vi "Correlation_Display.vi"(5 "Inst names":string[](array[string])=["HW 1", "HW 2"], 6 "OK":bool) -> (2 "correlation array":i32[][](array[numeric]) min=0 max=8)   [LabVIEW 2011]
uses:
  Globals/Meas_global.vi
panel:
  in  "number of correlation pairs":i32=1
  in  "correlation choices":i32[][](array[ring])=[[0, 1], [0, 0], [0, 0]] items=["LDA (U)", "LDA (W)", "XW (U) LDA Sync", "XW (W) LDA Sync", "RV (Sync)", "XW (U)", "XW (W)", "XW  U1", "XW  U2"]
  # "1st Pair"
  # "2nd Pair"
  # "3rd Pair"
  # "4th Pair"
  # "5th Pair"
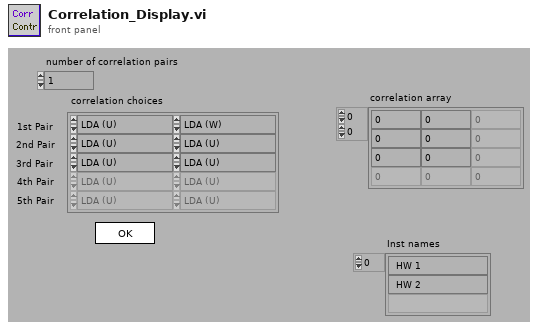
[diagram p1: front panel]
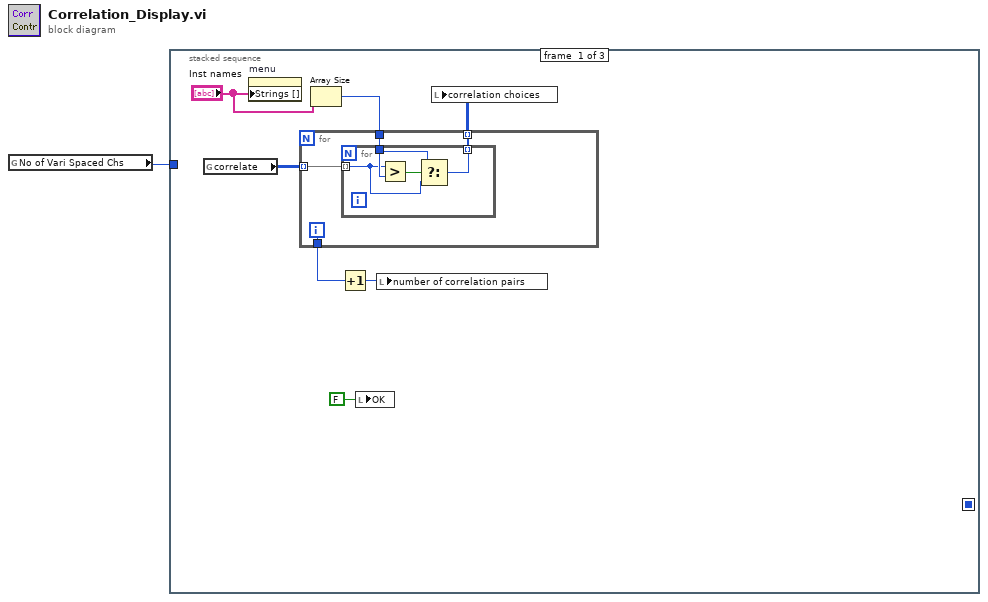
[diagram p0: block diagram]
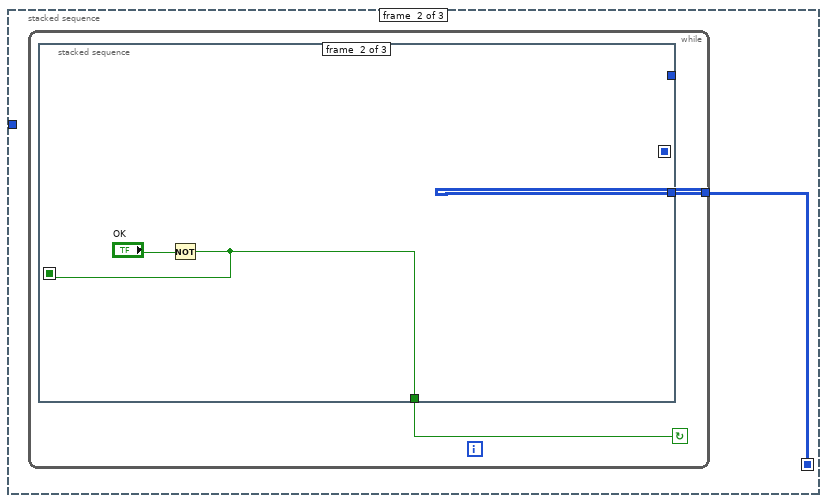
[diagram p2: hidden frame]
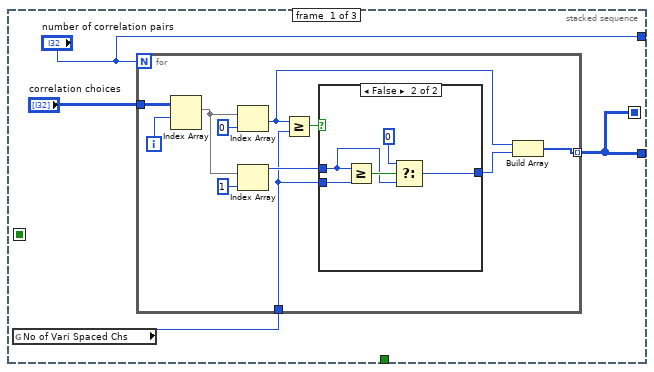
[diagram p3: hidden frame]
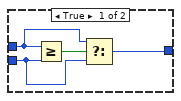
[diagram p4: hidden frame]
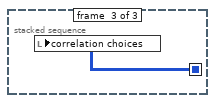
[diagram p5: hidden frame]
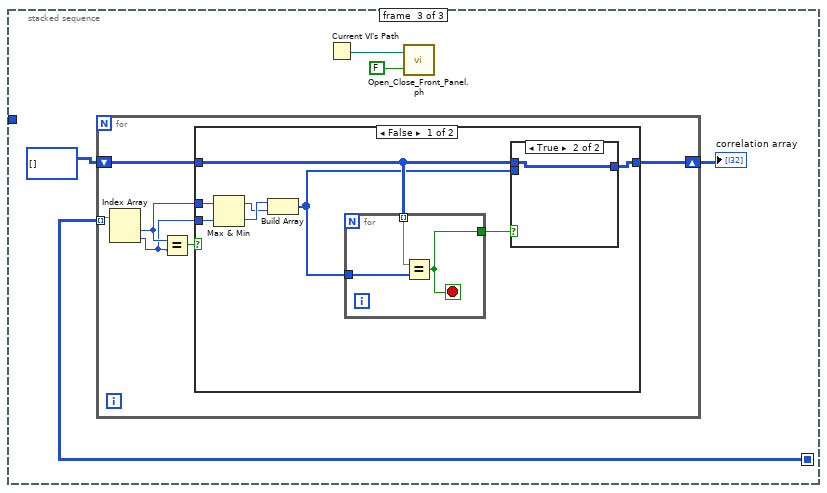
[diagram p6: hidden frame]
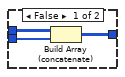
[diagram p7: hidden frame]
diagram:
  n1 = global read "Meas_global.vi" "No of Vari Spaced Chs"() -> (w1:i32)
  n2 = stacked-sequence {
    seq-local: [_ w17 _] -> [_ _ w49]
    tunnel: w1 -> [_ _ _]
    frame #0 {
      n3 = global read "Meas_global.vi" "correlate"() -> (w3:i32[][])
      n4 = property on="menu" class="Ring (strict)"("Strings []"="Inst names") -> ()  [unwired: 2 in, 2 out]
      n5 = Array Size(array="Inst names") -> (size(s)=w6:i32)
      n6 = for {
        tunnel: w6 -> [w12]
        tunnel: w3 -> [w11] mode=indexing
        tunnel: [w10] -> w7 mode=indexing
        tunnel: [w9] -> w5
        i -> [w9]
        n7 = for {
          tunnel: w12 -> [w15]
          tunnel: w11 -> [w14] mode=indexing
          tunnel: [w13] -> w10 mode=indexing
          n8 = Greater?(x=w14, y=w15) -> (0:w16:bool)
          n9 = Select(t=w15, s=w16, f=w14) -> (s? t:f=w13:i32)
        }
      }
      n10 = Increment(x=w5) -> (x+1=w4:i32)
      n11 = local write "OK"(FALSE ("OK")) -> ()
      n12 = local write "number of correlation pairs"(w4) -> ()
      n13 = local write "correlation choices"(w7) -> ()
    }
    frame #1 {
      n14 = while {
        tunnel: [w19] -> w17
        stop <- w18 continue-if-true
        n15 = stacked-sequence {
          seq-local: [w21 _ _] -> [_ _ w46]
          seq-local: [_ w44 _] -> [_ _ _]
          tunnel: [w21 _ _] -> w19
          tunnel: [_ w44 _] -> w18
          tunnel: ["number of correlation pairs" _ _] -> _
          frame #0 {
            n16 = global read "Meas_global.vi" "No of Vari Spaced Chs"() -> (w20:i32)
            n17 = for {
              N: "number of correlation pairs" -> [_]
              tunnel: "correlation choices" -> [w33]
              tunnel: w20 -> [w26]
              tunnel: [w28] -> w21 mode=indexing
              i -> [w34]
              n18 = Index Array(array=w33, index (row)=w34) -> (element=w30:i32[])  [unwired: 1 in]
              n19 = Index Array(array=w30, index=0 ("Index")) -> (element=w24:i32)
              n20 = Index Array(array=w30, index=1 ("Index")) -> (element=w27:i32)
              n21 = Greater Or Equal?(x=w24, y=w26) -> (x >= y?=w29:bool)
              n22 = case shown="False" w29 {
                tunnel: w27 -> [w37 w40]
                tunnel: w26 -> [w35 w41]
                tunnel: [w36 w42] -> w25
                frame True {
                  n23 = Greater Or Equal?(x=w37, y=w35) -> (x >= y?=w38:bool)
                  n24 = Select(t=w37, s=w38, f=w35) -> (s? t:f=w36:i32)
                }
                frame False {
                  n25 = Greater Or Equal?(x=w40, y=w41) -> (x >= y?=w43:bool)
                  n26 = Select(t=i8 0, s=w43, f=w40) -> (s? t:f=w42:i32)
                }
              }
              n27 = Build Array(w24, w25) -> (w28:i32[])
            }
          }
          frame #1 {
            n28 = Not(x="OK") -> (.not. x?=w44:bool)
          }
          frame #2 {
            n29 = local write "correlation choices"(w46) -> ()
          }
        }
      }
    }
    frame #2 {
      n30 = for {
        shift-right: [w56] -> w47
        shift-left: i32[][] [] -> [w57]
        tunnel: w49 -> [w54] mode=indexing
        n31 = Index Array(array=w54) -> (element #1=w53:i32, element #2=w52:i32)  [unwired: 2 in]
        n32 = Equal?(x=w53, y=w52) -> (x = y?=w55:bool)
        n33 = case shown="False" w55 {
          tunnel: w57 -> [w60 w73]
          tunnel: [w61 w73] -> w56
          tunnel: w53 -> [w65 _]
          tunnel: w52 -> [w64 _]
          frame False {
            n34 = Max & Min(x=w65, y=w64) -> (max(x,y)=w62:i32, min(x,y)=w63:i32)
            n35 = Build Array(w63, w62) -> (w59:i32[])
            n36 = for {
              tunnel: w60 -> [w72] mode=indexing
              tunnel: w59 -> [w71]
              tunnel: [w70] -> w58
              stop <- w70 stop-if-true
              n37 = Equal?(x=w72, y=w71) -> (x = y?=w70:bool)
            }
            n38 = case shown="True" w58 {
              tunnel: [w68 w69] -> w61
              tunnel: w60 -> [w67 w69]
              tunnel: w59 -> [w66 _]
              frame False {
                n39 = Build Array (concatenate)(w67, w66) -> (w68:i32[][])
              }
              frame True {
              }
            }
          }
          frame True {
          }
        }
      }
      "correlation array" <- w47
      n40 = Current VI's Path() -> (path=w51:path)
      n41 = call "Open_Close_Front_Panel.ph.vi"("Front Panel Window:Open"=FALSE, "VI path"=w51) -> ()  [unwired: 2 out]
    }
  }
